vi "test Import-Script-Deploy (Dynamic).vi"(8 "error in":errorcluster, 11 "Import-Script-Deploy.lvclass":refnum<class "Import-Script-Deploy.lvclass">) -> (0 "error out":errorcluster, 3 "Import-Script-Deploy.lvclass":refnum<class "Import-Script-Deploy.lvclass">)   [LabVIEW 2020, in "Import-Script-Deploy.lvclass"]
uses:
  Import-Script-Deploy.lvclass
  C:/Git/niveristand-custom-device-testing-tools/VeriStandTestCase/VeriStandTestCase.lvclass
  Shared/Device Parameters.ctl
  Shared/Initialization Method.ctl
  Import-Script-Deploy.lvclass/Import-Script-Deploy.ctl
  4b06c685-66bb-4135-9ad1-d89a50a95502.vi
  <vilib>/addons/_JKI Toolkits/VI Tester/TestCase.llb/TestCase.lvclass
  Scripting/Ballard/Ballard ARINC 429 Scripting.lvlib
  niveristand-custom-device-testing-tools/VeriStandTestUtilities/VeriStandTestUtilities.lvlib
  C:/Program Files (x86)/National Instruments/LabVIEW 2020/vi.lib/addons/_JKI Toolkits/VI Tester/TestCase.llb/TestCase.lvclass
  C:/Git/niveristand-ballard-arinc429-custom-device/Source/Custom Device Support/Tests/System/Import-Script-Deploy/Import-Script-Deploy.lvclass
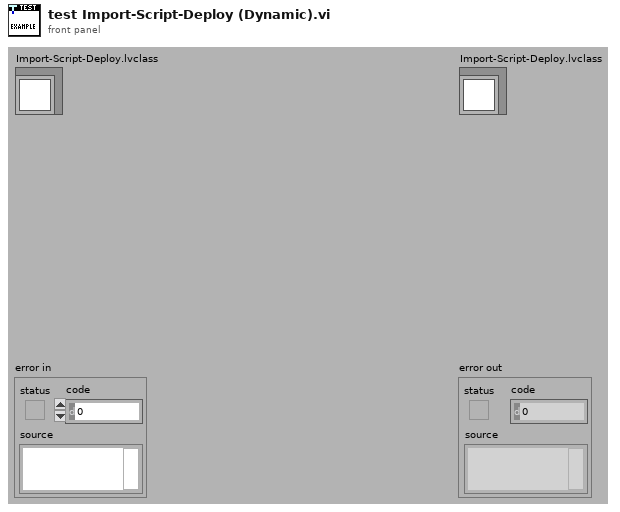
[diagram p1: front panel]
types:
  T1 = typedef "Device Parameters.ctl" = cluster{"initialization method":T2, "card number":i32, "PXI slot number":i32, "core number":i32}
  T2 = typedef "Initialization Method.ctl" = enum16{"PXI Slot Number", "Card Number"}
  T3 = typedef "Custom Device API.lvlib/Custom Device Item Ref.ctl" = u64
  T4 = typedef "NI_VS Workspace ExecutionAPI.lvlib/WorkspaceAPI.ctl" = refnum<k24>
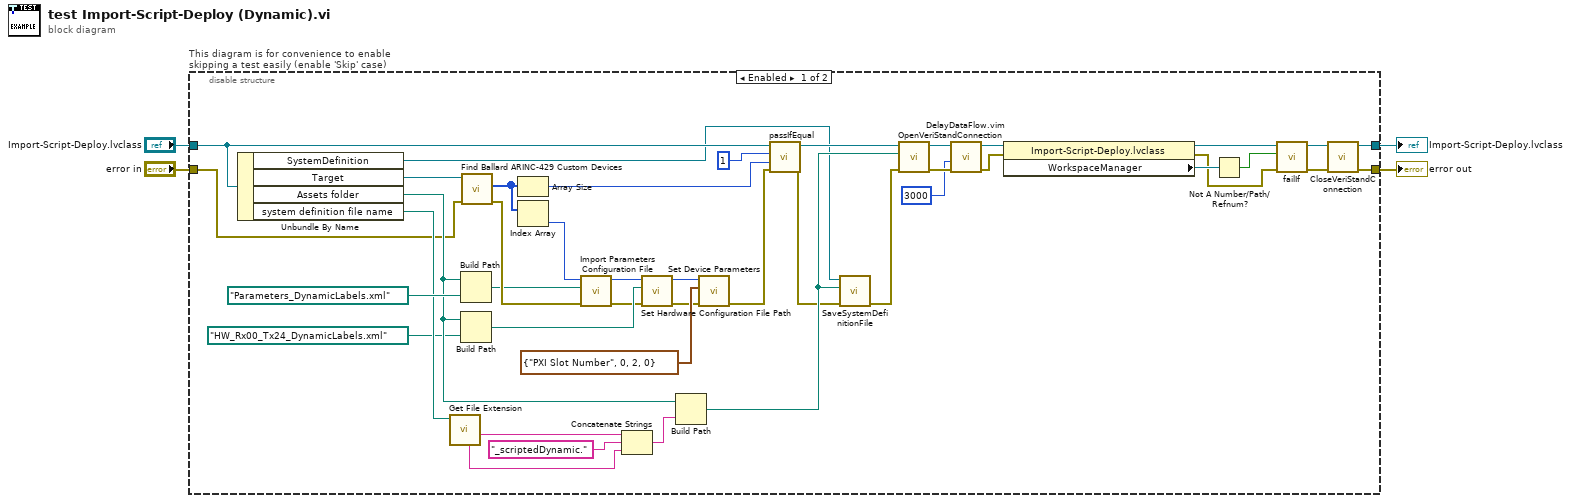
[diagram p0: block diagram]
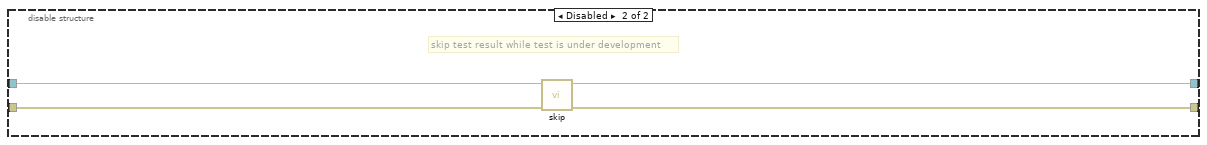
[diagram p2: hidden frame]
diagram:
  n1 = disable-structure "This diagram is for convenience to enable skipping a test easily (enable 'Skip' case)" shown="Enabled" {
    disable-tunnel: "Import-Script-Deploy.lvclass" -> [w35 w49]
    disable-tunnel: [w44 w48] -> w3
    disable-tunnel: "error in" -> [w11 w47]
    disable-tunnel: [w37 w46] -> w1
    frame Enabled {
      n2 = Unbundle By Name(w35) -> ("SystemDefinition"=w12:refnum<k24>, "Target"=w36:refnum<k24>, "Assets folder"=w18:path, "system definition file name"=w26:path)
      n3 = call <vilib>:"Get File Extension.vi"("file"=w26) -> ("filename without extension"=w25:string, "unmodified file extension"=w23:string)  [unwired: 6 in, 3 out]
      n4 = Build Path(base path=w18, name or relative path=path "Parameters_DynamicLabels.xml" ("Absolute or Relative Path")) -> (appended path=w5:path)
      n5 = Build Path(base path=w18, name or relative path=path "HW_Rx00_Tx24_DynamicLabels.xml" ("Absolute or Relative Path")) -> (appended path=w16:path)
      n6 = call "Find Ballard ARINC-429 Custom Devices.vi"("error in"=w11, "target in"=w36) -> ("error out"=w7:errorcluster, "Ballard ARINC 429 custom devices"=w10:u64[])  [unwired: 7 in, 1 out]
      n7 = Array Size(array=w10) -> (size(s)=w34:i32)
      n8 = Index Array(array=w10) -> (element=w6:u64)  [unwired: 1 in]
      n9 = call "Import Parameters Configuration File.vi"("error in"=w7, "parameters configuration file path"=w5, "Ballard ARINC 429 ref"=w6) -> ("error out"=w8:errorcluster, "Ballard ARINC 429 ref out"=w9:T3)  [unwired: 7 in]
      n10 = Concatenate Strings(w25, "_scriptedDynamic." ("string"), w23) -> (w22:string)
      n11 = call "Set Hardware Configuration File Path.vi"("error in"=w8, "path"=w16, "custom device ref"=w9) -> ("error out"=w14:errorcluster, "custom device ref out"=w15:T3)  [unwired: 7 in]
      n12 = Build Path(base path=w18, name or relative path=w22) -> (appended path=w21:path)
      n13 = call "Set Device Parameters.vi"("error in"=w14, "device parameters"=T1 {"initialization method"=enum."PXI Slot Number", "card number"=0, "PXI slot number"=2, "core number"=0}, "Ballard ARINC 429 custom device in"=w15) -> ("error out"=w13:errorcluster)  [unwired: 7 in, 1 out]
      n14 = call-dynamic "passIfEqual.vi"("error in (no error)"=w13, "y"=w34, "x"=1 ("size(s)"), "TestCase in"=w35) -> ("error out"=w19:errorcluster, "TestCase out"=w32:refnum<class "Import-Script-Deploy.lvclass">)  [unwired: 6 in]
      n15 = call "SaveSystemDefinitionFile.vi"("error in (no error)"=w19, "System Definition File in"=w21, "System Definition Reference in"=w12) -> ("error out"=w20:errorcluster)  [unwired: 7 in, 1 out]
      n16 = call-dynamic "OpenVeriStandConnection.vi"("error in (no error)"=w20, "System Definition File"=w21, "VeriStand Test Case in"=w32) -> ("error out"=w31:errorcluster, "VeriStand Test Case out"=w30:refnum<class "Import-Script-Deploy.lvclass">)  [unwired: 6 in, 1 out]
      n17 = call "DelayDataFlow.vim"("value in"=w31, "milliseconds to wait"=u32 3000) -> ("value out"=w45:errorcluster)  [unwired: 2 in, 1 out]
      n18 = property class="Import-Script-Deploy.lvclass"(reference=w30, error in=w45) -> (reference out=w43:refnum<class "Import-Script-Deploy.lvclass">, error out=w38:errorcluster, "WorkspaceManager"=w40:T4)
      n19 = Not A Number/Path/Refnum?(number/path/refnum=w40) -> (NaN/Path/Refnum?=w39:bool)
      n20 = call-dynamic "failIf.vi"("error in (no error)"=w38, "fail"=w39, "TestCase in"=w43) -> ("error out"=w41:errorcluster, "TestCase out"=w42:refnum<class "Import-Script-Deploy.lvclass">)  [unwired: 7 in]
      n21 = call-dynamic "CloseVeriStandConnection.vi"("error in (no error)"=w41, "VeriStand Test Case in"=w42) -> ("error out"=w44:errorcluster, "VeriStand Test Case out"=w37:refnum<class "Import-Script-Deploy.lvclass">)  [unwired: 8 in]
    }
    frame Disabled {
      # "skip test result while test is under development"
      n22 = call <vilib>:"skip.vi"("error in (no error)"=w47, "TestCase in"=w49) -> ("error out"=w48:errorcluster, "TestCase out"=w46:refnum<class "Import-Script-Deploy.lvclass">)  [unwired: 8 in]
    }
  }
  "error out" <- w3
  "Import-Script-Deploy.lvclass" <- w1
